vi "FindIndex(SubVI).vi"(8 "Error In":errorcluster, 10 "Name":string, 11 "Strings And Values[]":cluster{"String":string, "Value":string}[](array[cluster])) -> (0 "Error Out":errorcluster, 3 "Index":dbl)   [LabVIEW 2018]
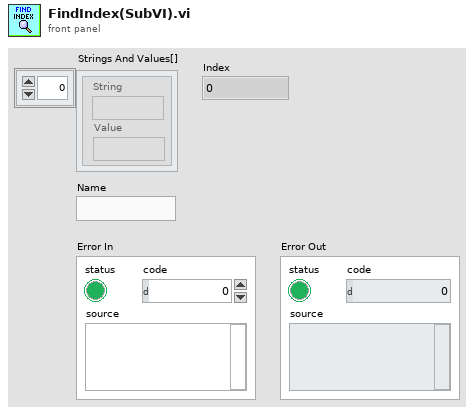
[diagram p1: front panel]
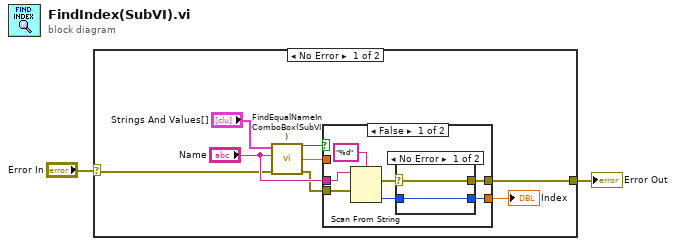
[diagram p0: block diagram]
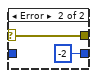
[diagram p2: hidden frame]
diagram:
  n1 = case shown="No Error" "Error In" {
    selector: "Error In" -> [w5 w24]
    tunnel: [w3 w24] -> w1
    frame No Error {
      n2 = call "FindEqualNameInComboBox(SubVI).vi"("Error In"=w5, "Name"="Name", "Strings And Values[]"="Strings And Values[]") -> ("Error Out"=w4:errorcluster, "NumPlot"=w9:dbl, "Does the array contain this name?"=w7:bool)  [unwired: 6 in]
      n3 = case shown="False" w7 {
        tunnel: "Name" -> [w16 _]
        tunnel: w9 -> [_ w23]
        tunnel: [w13 w23] -> w10
        tunnel: w4 -> [w12 w22]
        tunnel: [w11 w22] -> w3
        frame False {
          n4 = Scan From String(format string="%d", input string=w16, error in=w12) -> (error out=w15:errorcluster, output 1=w14:i32)  [unwired: 2 in, 2 out]
          n5 = case shown="No Error" w15 {
            selector: w15 -> [w18 w20]
            tunnel: w14 -> [w19 _]
            tunnel: [w19 -2] -> w13
            tunnel: [w18 w20] -> w11
            frame No Error {
            }
            frame Error {
            }
          }
        }
        frame True {
        }
      }
      "Index" <- w10
    }
    frame Error {
    }
  }
  "Error Out" <- w1
